vi "LVJSON List.vi"(8 "error in (no error)":errorcluster, 11 "Root Element in":T2) -> (0 "error out":errorcluster, 1 "Type":T1, 2 "Keys/Indexes":string[](array[string]), 3 "dup Root Element":T2)   [LabVIEW 2019, in "labview_json.lvlib"]
uses:
  labview_json.lvlib
  Element.ctl
  Element Type.ctl
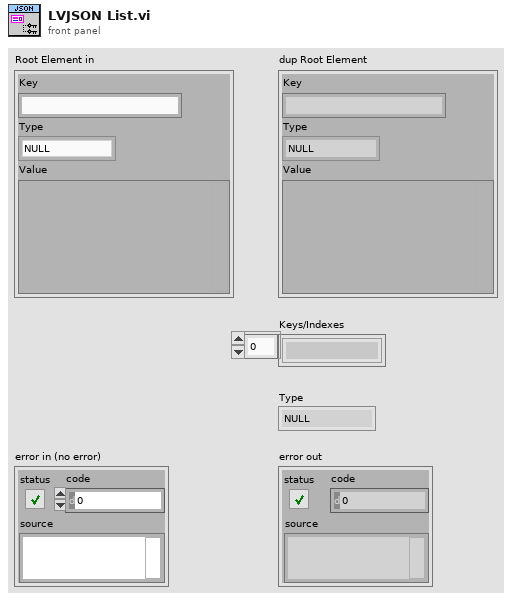
[diagram p1: front panel]
types:
  T1 = typedef "labview_json.lvlib/Element Type.ctl" = enum8{"NULL", "OBJECT", "ARRAY", "BOOL", "INT", "UINT", "FLOAT", "STRING"}
  T2 = typedef "labview_json.lvlib/Element.ctl" = cluster{"Key":string, "Type":T1, "Value":variant}
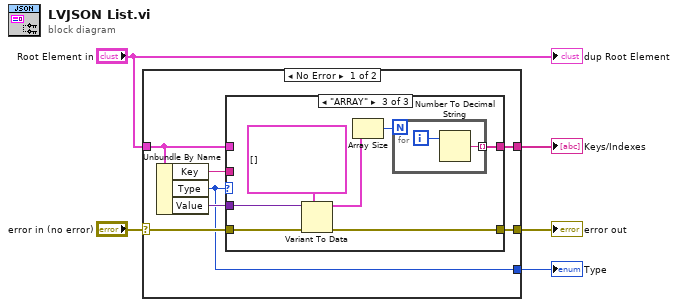
[diagram p0: block diagram]
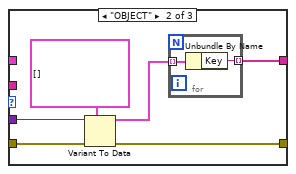
[diagram p3: hidden frame]
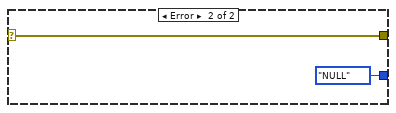
[diagram p4: hidden frame]
diagram:
  n1 = case shown="No Error" "error in (no error)" {
    selector: "error in (no error)" -> [w12 w32]
    tunnel: [w11 w32] -> w4
    tunnel: [w10 _] -> w1
    tunnel: "Root Element in" -> [w9 _]
    tunnel: [w6 Element_Type."NULL" ("Type")] -> w2
    frame No Error {
      n2 = Unbundle By Name(w9) -> ("Key"=w7:string, "Type"=w6:T1, "Value"=w8:variant)
      n3 = case shown="\"ARRAY\"" w6 {
        tunnel: w8 -> [_ w19 w28]
        tunnel: w7 -> [_ _ _]
        tunnel: w12 -> [w13 w17 w26]
        tunnel: [w13 w16 w25] -> w11
        tunnel: [_ w14 w24] -> w10
        tunnel: w9 -> [_ _ _]
        frame "NULL", "BOOL".."STRING" {
        }
        frame "OBJECT" {
          n4 = Variant To Data(error in=w17, type=T2[] [] ("Values"), Variant=w19) -> (data=w15:T2[], error out=w16:errorcluster)
          n5 = for {
            tunnel: w15 -> [w21] mode=indexing
            tunnel: [w20] -> w14 mode=indexing
            n6 = Unbundle By Name(w21) -> ("Key"=w20:string)
          }
        }
        frame "ARRAY" {
          n7 = Variant To Data(error in=w26, type=T2[] [] ("Values"), Variant=w28) -> (data=w23:T2[], error out=w25:errorcluster)
          n8 = Array Size(array=w23) -> (size(s)=w22:i32)
          n9 = for {
            N: w22 -> [_]
            tunnel: [w29] -> w24 mode=indexing
            i -> [w30]
            n10 = Number To Decimal String(number=w30) -> (decimal integer string=w29:string)  [unwired: 1 in]
          }
        }
      }
    }
    frame Error {
    }
  }
  "error out" <- w4
  "Keys/Indexes" <- w1
  "Type" <- w2
  "dup Root Element" <- "Root Element in"
